vi "Parse DAT String.vi"(8 "error in (no error)":errorcluster, 11 "spreadsheet string":string[][](array[string])) -> (0 "error out":errorcluster, 2 "Notes":string, 3 "Data (Dictionary)":T1[](array[typedef]))   [LabVIEW 2016, in "Data.DAT.lvclass"]
uses:
  Data.DAT.lvclass
  Data/Typedefs/Dictionary--cluster.ctl
  Data/Data.lvclass
panel:
  in  "header length":i32=11
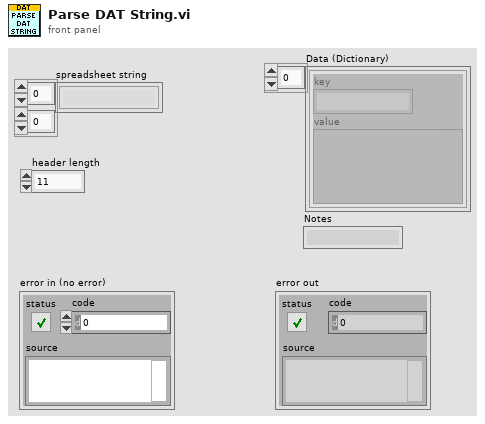
[diagram p1: front panel]
types:
  T1 = typedef "Data.lvclass/Dictionary--cluster.ctl" = cluster{"key":string, "value":variant}
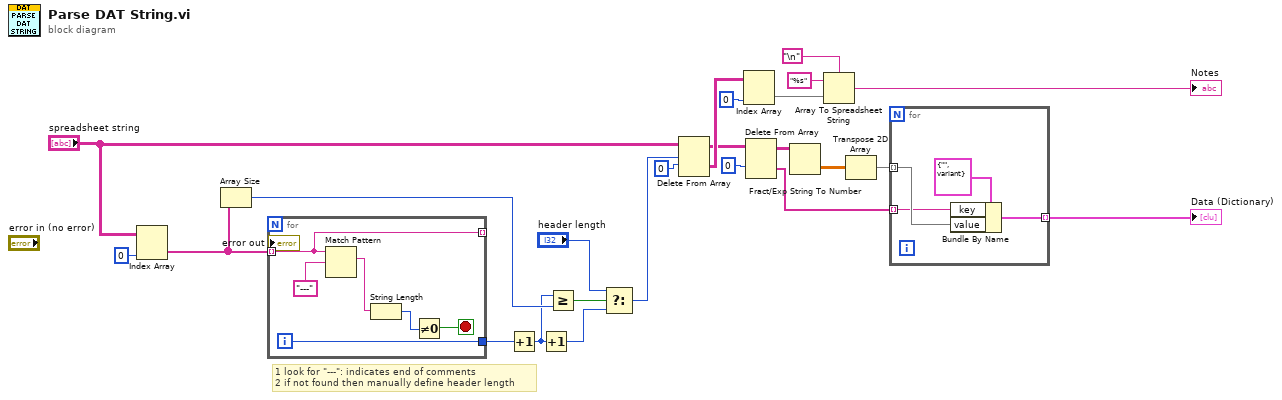
[diagram p0: block diagram]
diagram:
  # "1 look for \"---\": indicates end of comments\n2 if not found then manually define header length"
  n1 = Index Array(array="spreadsheet string", index (col)=0 ("disabled index (col)")) -> (element=w13:string[])  [unwired: 1 in]
  n2 = Array Size(array=w13) -> (size(s)=w16:i32)
  n3 = for {
    tunnel: w13 -> [w25] mode=indexing
    tunnel: [w26] -> w12
    tunnel: [w25] -> _ mode=indexing
    i -> [w26]
    stop <- w28 stop-if-true
    n4 = Match Pattern(string=w25, regular expression="---") -> (match substring=w29:string)  [unwired: 4 out]
    n5 = String Length(string=w29) -> (length=w27:i32)
    n6 = Not Equal To 0?(x=w27) -> (x != 0?=w28:bool)
  }
  n7 = Increment(x=w12) -> (x+1=w14:i32)
  n8 = Increment(x=w14) -> (x+1=w17:i32)
  n9 = Greater Or Equal?(x=w14, y=w16) -> (x >= y?=w15:bool)
  n10 = Select(t="header length", s=w15, f=w17) -> (s? t:f=w19:i32)
  n11 = Delete From Array(array="spreadsheet string", length=w19, index (row)=0) -> (deleted portion=w8:string[][], array with subset deleted=w4:string[][])  [unwired: 1 in]
  n12 = Index Array(array=w8, index (col)=0 ("disabled index (col)")) -> (element=w9:string[])  [unwired: 1 in]
  n13 = Delete From Array(array=w4, index (row)=0) -> (deleted portion=w20:string[], array with subset deleted=w3:string[][])  [unwired: 2 in]
  n14 = Fract/Exp String To Number(string=w3) -> (number=w21:dbl[][])  [unwired: 3 in, 1 out]
  n15 = Array To Spreadsheet String(delimiter (Tab)="\n", array=w9, 3:"%s" ("format string")) -> (spreadsheet string=→"Notes":string)
  n16 = Transpose 2D Array(2D array=w21) -> (transposed array=w22:dbl[][])
  n17 = for {
    tunnel: w20 -> [w31] mode=indexing
    tunnel: w22 -> [w32] mode=indexing
    tunnel: [w34] -> w23 mode=indexing
    n18 = Bundle By Name(cluster=T1 {"key"="", "value"=variant} ("key-value"), "key"=w31, "value"=w32) -> (w34:T1)
  }
  "Data (Dictionary)" <- w23
